vi "Endpoint Configuration Page.vi"(8 "error in (no error)":errorcluster, 11 "Node Ptr":T4 format="%.0x") -> (0 "error out":errorcluster)   [LabVIEW 2017, in "SLSC Switch System Explorer.lvlib"]
uses:
  SLSC Switch System Explorer.lvlib
  <vilib>/NI Veristand/Custom Device API/Custom Device Item Ref.ctl
  Channel.ctl
  Channel Type.ctl
  Shared/UI Common/Sort Button.ctl
  Endpoint Configuration Page Controls.ctl
  16100924-b29d-4153-bcd0-e39b01036c8d.vi
  16100924-b29d-4153-bcd0-e39b01036c8d.vi/6b8804ba-2cd8-479f-80f9-0d8a68c2bdc7.vi
  16100924-b29d-4153-bcd0-e39b01036c8d.vi/77c8236f-6af0-4988-9b27-3d2302fd99e7.vi
  <vilib>/NI Veristand/Custom Device API/Custom Device API.lvlib
  Shared/UI Common/UI Common.lvlib
panel:
  in  "Sort":T1
  out "Configuration":string="Configuration"
  out "Endpoint":string="Endpoint"
  in  "Channels":T2[](array[typedef])
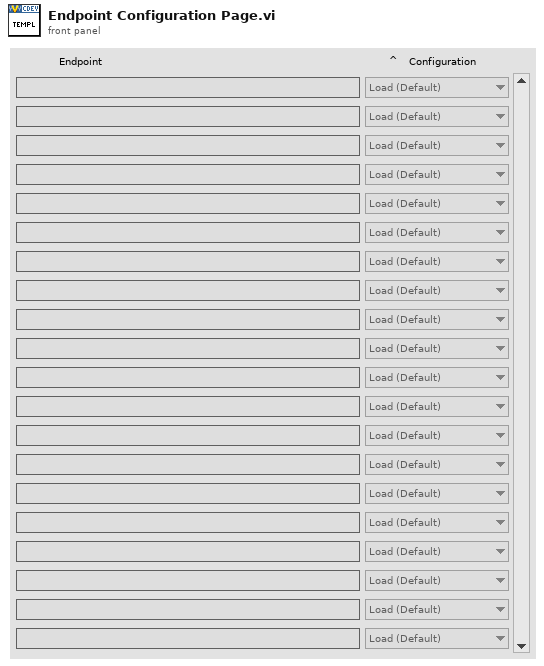
[diagram p1: front panel]
types:
  T1 = typedef "UI Common.lvlib/Sort Button.ctl" = bool
  T2 = typedef "SLSC Switch System Explorer.lvlib/Channel.ctl" = cluster{"Endpoint":string, "Configuration":T3}
  T3 = typedef "SLSC Switch System Explorer.lvlib/Channel Type.ctl" = enum16{"Load (Default)", "Source", "Configuration"}
  T4 = typedef "Custom Device API.lvlib/Custom Device Item Ref.ctl" = u64
  T5 = typedef "SLSC Switch System Explorer.lvlib/Endpoint Configuration Page Controls.ctl" = cluster{"Channels":refnum<vi>, "Endpoint Label":refnum<vi>, "Configuration Label":refnum<vi>, "Sort":refnum<vi>}
  T6 = typedef "Custom Device API.lvlib/Custom Device Commands.ctl" = enum16{"Default", "Item renamed", "Shutdown", "Dynamic button pressed"}
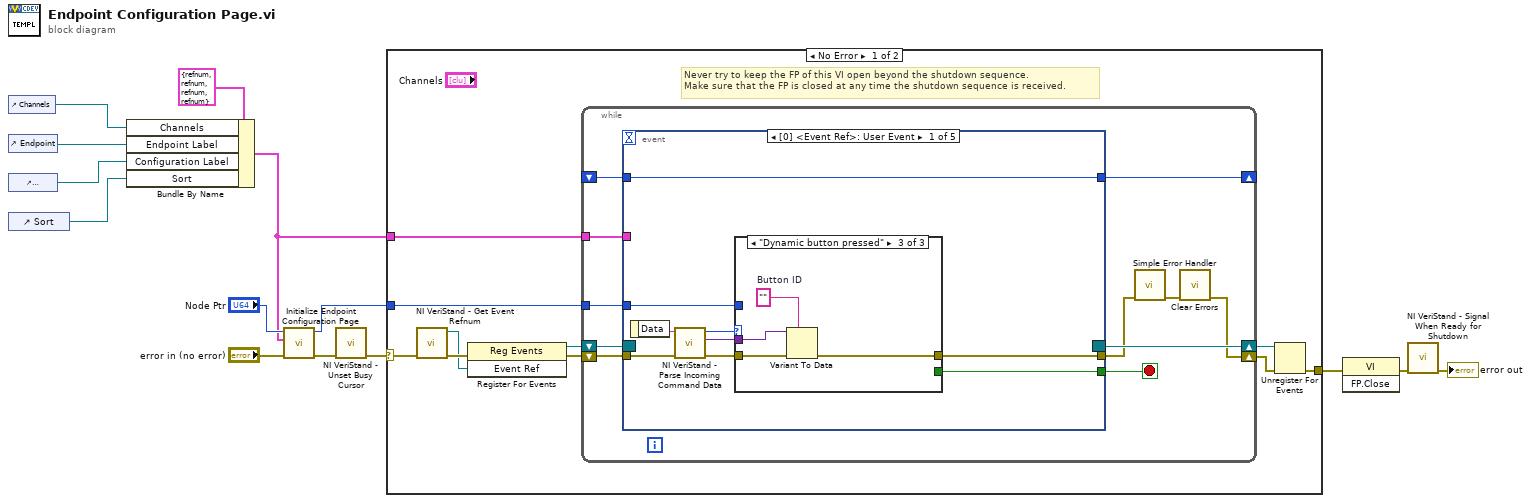
[diagram p0: block diagram]
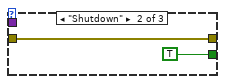
[diagram p3: hidden frame]
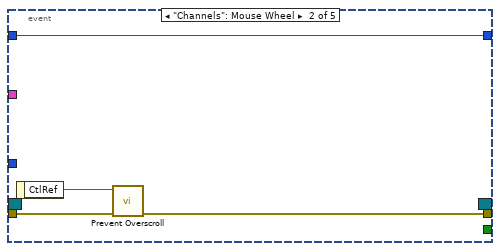
[diagram p4: hidden frame]
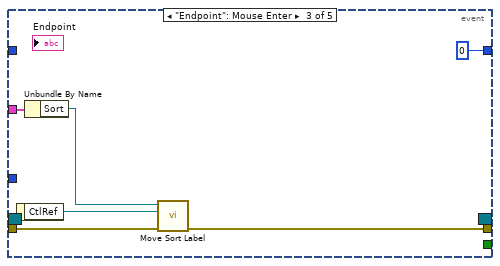
[diagram p5: hidden frame]
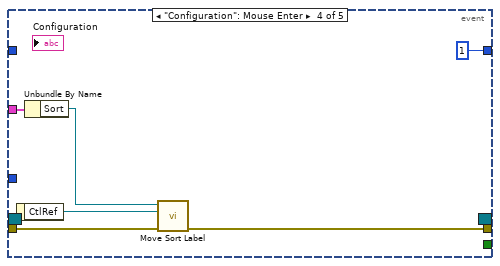
[diagram p6: hidden frame]
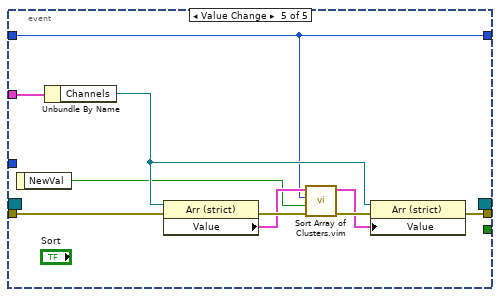
[diagram p7: hidden frame]
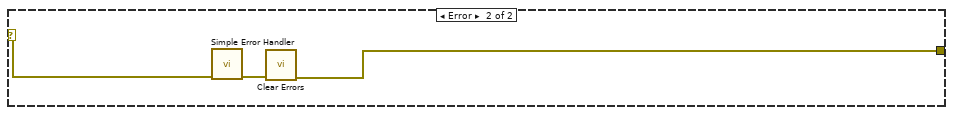
[diagram p8: hidden frame]
diagram:
  n1 = control-ref of="Channels"() -> (w7:refnum<vi>)
  n2 = control-ref of="Endpoint"() -> (w6:refnum<vi>)
  n3 = control-ref of="Configuration"() -> (w5:refnum<vi>)
  n4 = control-ref of="Sort"() -> (w4:refnum<vi>)
  n5 = Bundle By Name(cluster=T5 {"Channels"=refnum, "Endpoint Label"=refnum, "Configuration Label"=refnum, "Sort"=refnum} ("Endpoint Configuration Page Controls"), "Channels"=w7, "Endpoint Label"=w6, "Configuration Label"=w5, "Sort"=w4) -> (w3:T5)
  n6 = call "Initialize Endpoint Configuration Page.vi"("error in (no error)"="error in (no error)", "Endpoint Configuration Page Controls"=w3, "Node Ptr"="Node Ptr") -> ("error out"=w2:errorcluster, "Endpoint Configuration Section Ref out"=w9:T4)  [unwired: 7 in]
  n7 = call <vilib>:"NI VeriStand - Unset Busy Cursor.vi"("error in (no error)"=w2) -> ("error out"=w12:errorcluster)  [unwired: 10 out]
  n8 = case shown="No Error" w12 {
    selector: w12 -> [w19 w80]
    tunnel: [w22 w78] -> w14
    tunnel: w9 -> [w20 _]
    tunnel: w3 -> [w17 _]
    frame No Error {
      # "Never try to keep the FP of this VI open beyond the shutdown sequence.\nMake sure that the FP is closed at any time the shutdown sequence is received."
      n9 = call <vilib>:"NI VeriStand - Get Event Refnum.vi"("error in (no error)"=w19) -> ("error out"=w16:errorcluster, "Event Ref"=w15:refnum<user-event>)  [unwired: 9 out]
      n10 = register-events(error in=w16, w15) -> (reference out=w21:refnum<event-registration>, error out=w18:errorcluster)  [unwired: 1 in]
      n11 = while {
        tunnel: w20 -> [w31]
        shift-right: [w28] -> w23
        shift-left: w18 -> [w34]
        shift-right: [w35] -> w24
        shift-left: w21 -> [w33]
        shift-right: [w27] -> _
        shift-left: _ -> [w25]
        tunnel: w17 -> [w26]
        stop <- w32 stop-if-true
        n12 = event shown="[0] <Event Ref>: User Event" {
          selector: w33 -> [_ _ _ _ _]
          dyn-events: [_ _ _ _ _] -> w35
          timeout: _ -> [_ _ _ _ _]
          tunnel: w34 -> [w44 w55 w61 w67 w77]
          tunnel: [w40 _ _ _ _] -> w32
          tunnel: [w39 w54 w60 w66 w72] -> w30
          tunnel: w31 -> [w38 _ _ _ _]
          tunnel: [w36 w52 0 ("index of element") 1 ("index of element") w68] -> w27
          tunnel: w26 -> [_ _ w57 w63 w76]
          tunnel: w25 -> [w36 w52 _ _ w68]
          event User Event {
            n13 = event-data() -> ("Data"=w43:string)  [unwired: 1 out]
            n14 = call <vilib>:"NI VeriStand - Parse Incoming Command Data.vi"("error in (no error)"=w44, "Incoming data"=w43) -> ("error out"=w42:errorcluster, "Outgoing data"=w37:variant, "Action"=w41:T6)  [unwired: 7 out]
            n15 = case shown="\"Dynamic button pressed\"" w41 {
              tunnel: w42 -> [w45 w46 w51]
              tunnel: [_ TRUE _] -> w40
              tunnel: [w45 w46 w48] -> w39
              tunnel: w38 -> [_ _ _]
              tunnel: w37 -> [_ _ w50]
              frame "Default", Default {
              }
              frame "Shutdown" {
              }
              frame "Dynamic button pressed" {
                w49 = ""  # Button ID
                n16 = Variant To Data(error in=w51, type=w49, Variant=w50) -> (error out=w48:errorcluster)  [unwired: 1 out]
              }
            }
          }
          event "Channels": Mouse Wheel {
            n17 = event-data() -> ("CtlRef"=w53:refnum<vi>)  [unwired: 1 out]
            n18 = call "Prevent Overscroll.vi"("error in (no error)"=w55, "Array Refnum"=w53) -> ("error out"=w54:errorcluster)  [unwired: 8 in, 1 out]
          }
          event "Endpoint": Mouse Enter {
            n19 = event-data() -> ("CtlRef"=w59:refnum<vi>)  [unwired: 1 out]
            n20 = Unbundle By Name(w57) -> ("Sort"=w56:refnum<vi>)
            n21 = call "Move Sort Label.vi"("error in (no error)"=w61, "Target Label"=w59, "Sort"=w56) -> ("error out"=w60:errorcluster)  [unwired: 8 in]
          }
          event "Configuration": Mouse Enter {
            n22 = event-data() -> ("CtlRef"=w65:refnum<vi>)  [unwired: 1 out]
            n23 = Unbundle By Name(w63) -> ("Sort"=w62:refnum<vi>)
            n24 = call "Move Sort Label.vi"("error in (no error)"=w67, "Target Label"=w65, "Sort"=w62) -> ("error out"=w66:errorcluster)  [unwired: 8 in]
          }
          event Value Change {
            n25 = event-data() -> ("NewVal"=w69:T1)  [unwired: 1 out]
            n26 = Unbundle By Name(w76) -> ("Channels"=w70:refnum<vi>)
            n27 = property class="Arr (strict)"(reference=w70, error in=w77) -> (error out=w75:errorcluster, "Value"=w74:T2[])  [unwired: 1 out]
            n28 = call "Sort Array of Clusters.vim"("error in (no error)"=w75, "Descending"=w69, "index"=w68, "Array"=w74) -> ("error out"=w73:errorcluster, "Sorted Array"=w71:T2[])  [unwired: 6 in]
            n29 = property class="Arr (strict)"(reference=w70, error in=w73, "Value"=w71) -> (error out=w72:errorcluster)  [unwired: 1 out]
          }
        }
        n30 = call <vilib>:"Simple Error Handler.vi"("error in (no error)"=w30) -> ("error out"=w29:errorcluster)  [unwired: 1 in, 7 out]
        n31 = call <vilib>:"Clear Errors.vi"("error in (no error)"=w29) -> ("error out"=w28:errorcluster)  [unwired: 1 in, 5 out]
      }
      n32 = Unregister For Events(event registration refnum=w24, error in=w23) -> (error out=w22:errorcluster)
    }
    frame Error {
      n33 = call <vilib>:"Simple Error Handler.vi"("error in (no error)"=w80) -> ("error out"=w79:errorcluster)  [unwired: 1 in, 7 out]
      n34 = call <vilib>:"Clear Errors.vi"("error in (no error)"=w79) -> ("error out"=w78:errorcluster)  [unwired: 1 in, 5 out]
    }
  }
  n35 = invoke class="VI" method="FP.Close"(error in=w14) -> (error out=w1:errorcluster)  [unwired: 2 in, 2 out]
  n36 = call <vilib>:"NI VeriStand - Signal When Ready for Shutdown.vi"("error in (no error)"=w1) -> ("error out"=→"error out":errorcluster)  [unwired: 10 out]
